vi "Agilent 34970 Setup Temperature HEWH.vi"(10 "Agilent Channel Input":string="111,112,113,114,115,116,109,110,201,202,203,204,205,206,207,208,209,210,211,212,213,214,215,216,107,108,301,302,303,304,305,306,307,308,309,310,311,312,313,314,315,316,105,106", 11 "VISA Refnum in":refnum<visa-resource-name>) -> ()   [LabVIEW 2016]
uses:
  Agilent 34970.lvlib
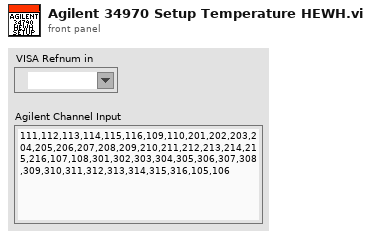
[diagram p1: front panel]
types:
  T1 = cluster{"Thermocouple Type (Last)":enum16{"B", "E", "J", "K", "N", "R", "S", "T", "Default (Last)"}, "TC Rjunction (2:Int)":enum16{"Fixed", "External", "Internal"}, "Fixed Rjunction Temp (0:Manual)":enum16{"Manual", "Minimum", "Maximum"}, "TC Auto Check? (F:Don't Check)":bool, "Rjunct Temp Value (0)":dbl}
  T2 = enum16{"Thermocouple", "Thermistor", "RTD", "4-Wire RTD"}
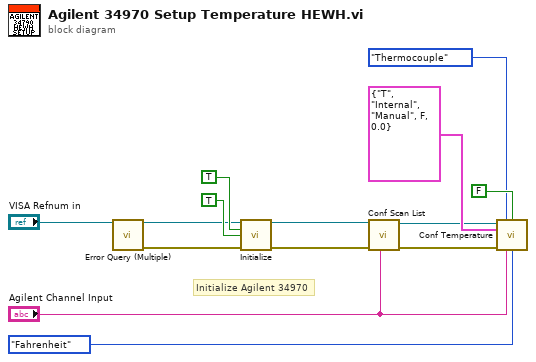
[diagram p0: block diagram]
diagram:
  # "Initialize Agilent 34970"
  n1 = call "Error Query (Multiple).vi"("VISA Resource Name"="VISA Refnum in") -> ("VISA Resource Name Out"=w8:refnum<visa-resource-name>, "error out"=w9:errorcluster)  [unwired: 11 in, 2 out]
  n2 = call "Initialize.vi"("VISA Resource Name"=w8, "ID Query (T: Check)"=TRUE, "Reset (T: Reset)"=TRUE, "error in (no error)"=w9) -> ("VISA Resource Name Out"=w13:refnum<visa-resource-name>, "error out"=w14:errorcluster)  [unwired: 10 in]
  n3 = call "Conf Scan List.vi"("Scan List (empty)"="Agilent Channel Input", "error in (no error)"=w14, "VISA Resource Name"=w13) -> ("error out"=w1:errorcluster, "VISA Resource Name Out"=w2:refnum<visa-resource-name>)  [unwired: 6 in, 1 out]
  n4 = call "Conf Temperature.vi"("VISA Resource Name"=w2, "Transducer Type (0:TC)"=T2."Thermocouple", "Set/Check? (F:Set)"=FALSE, "Thermocouple Configuration"=T1 {"Thermocouple Type (Last)"=enum."T", "TC Rjunction (2:Int)"=enum."Internal", "Fixed Rjunction Temp (0:Manual)"=enum."Manual", "TC Auto Check? (F:Don't Check)"=FALSE, "Rjunct Temp Value (0)"=0.0}, "error in (no error)"=w1, "Channel List(empty)"="Agilent Channel Input", "Units (0:Celsius)"=enum16{"Celsius", "Fahrenheit", "Kelvin"}."Fahrenheit") -> ()  [unwired: 6 in, 3 out]
